vi "SbigDecodeString.vi"(1 "Array of U16":u16[](array[numeric])) -> (0 "String":string)   [LabVIEW 2009]
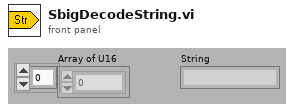
[diagram p1: front panel]
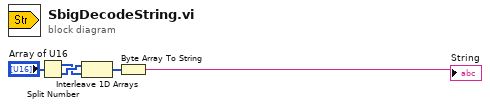
[diagram p0: block diagram]
diagram:
  n1 = Split Number(x="Array of U16") -> (hi(x)=w4:u8[], lo(x)=w5:u8[])
  n2 = Interleave 1D Arrays(w5, w4) -> (w3:u8[])
  n3 = Byte Array To String(unsigned byte array=w3) -> (string=→"String":string)
